vi "KeyboardSimulation_Tests.vi"(11 "error in":errorcluster) -> (15 "error out":errorcluster)   [LabVIEW 2016, in "DronaTest.lvlib"]
uses:
  DronaTest.lvlib
  APIs/Stimulus/KeyBoardSimulation/typedef/VirtualKey.ctl
  APIs/Stimulus/KeyBoardSimulation/typedef/Action.ctl
  APIs/Stimulus/KeyBoardSimulation/KeyBoardSimulationForTargetVI.vi
  APIs/Assert/AssertControlValue/Equal.vi
  <vilib>/addons/_JKI Toolkits/Caraya/classes/Test/Test.lvclass
  Drona.lvlib
  APIs/Stimulus/KeyBoardSimulation/KeyboardSimulation.lvlib
  APIs/Assert/AssertControlValue/AssertControlValue.lvlib
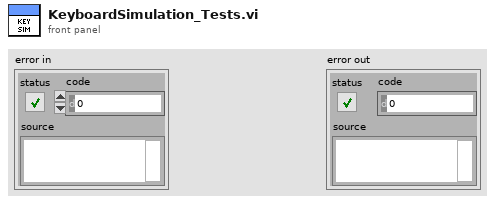
[diagram p1: front panel]
types:
  T1 = typedef "Drona.lvlib/KeyboardSimulation.lvlib/VirtualKey.ctl" = u8
  T2 = typedef "Drona.lvlib/KeyboardSimulation.lvlib/Action.ctl" = enum16{"Press", "Up", "Down"}
  T3 = cluster{" Key":T1, "Action":T2, "Delay (ms)":u32}[]
  T4 = enum16{"TypeHello_ControlValueShouldBeHello", "AddStringToClipboardAndPaste_ControlValueShouldBeStringFromClipboard", "TypeNegative25_ControlValueShouldBeNegative25", "Type255_ControlValueCoerceTo100", "TypeNegative257_ControlValueCoerceToNegative100"}[]
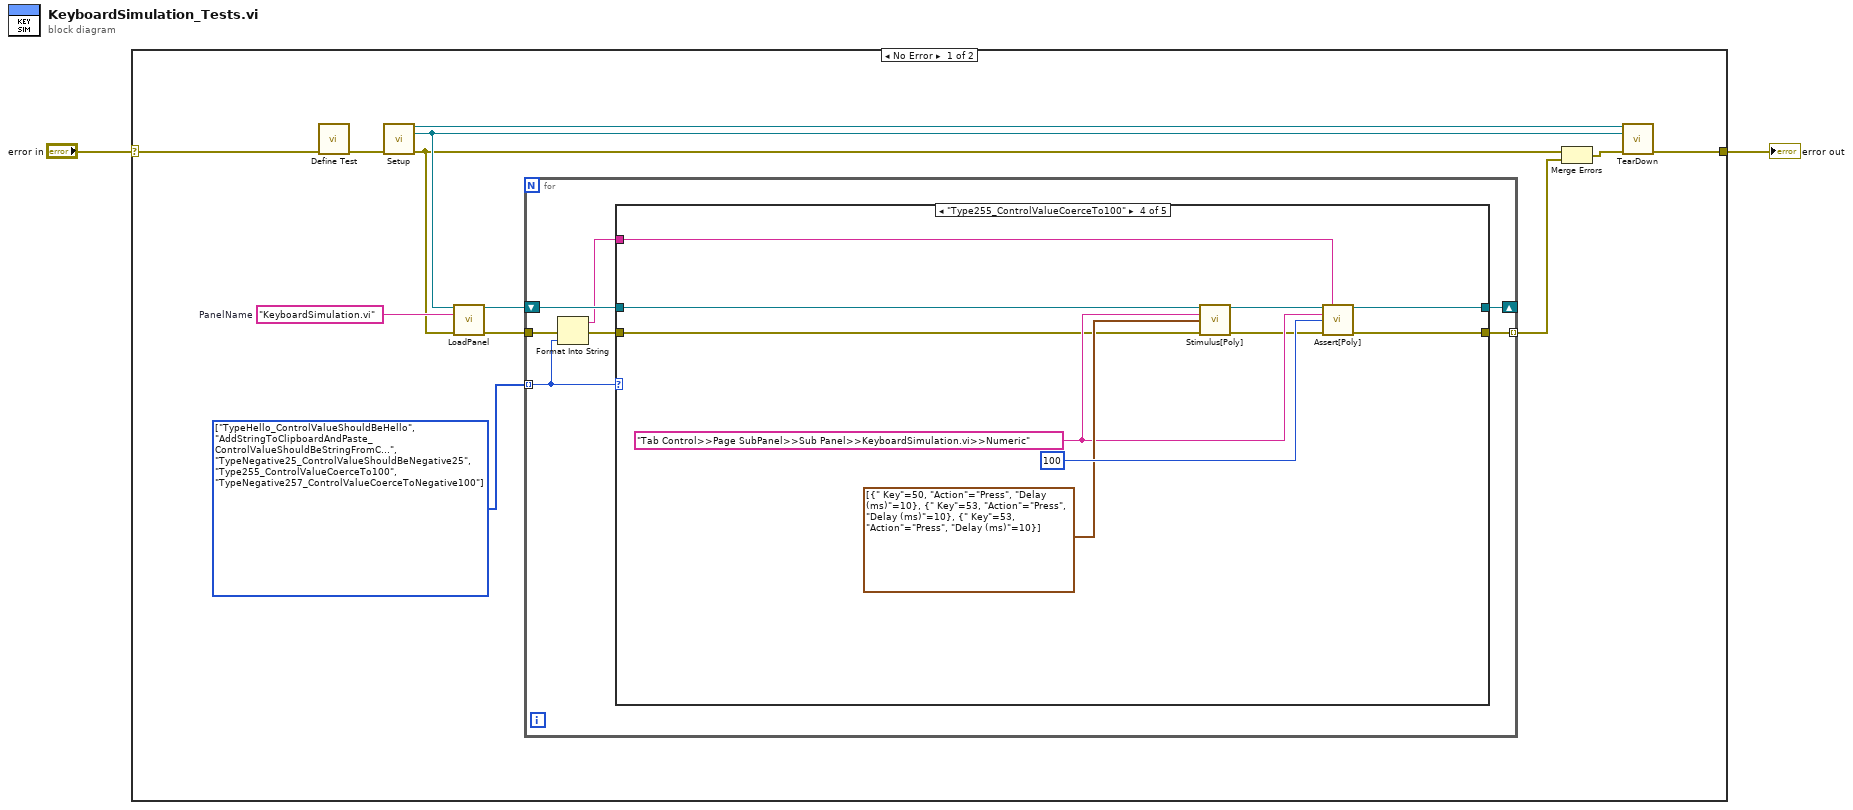
[diagram p0: block diagram]
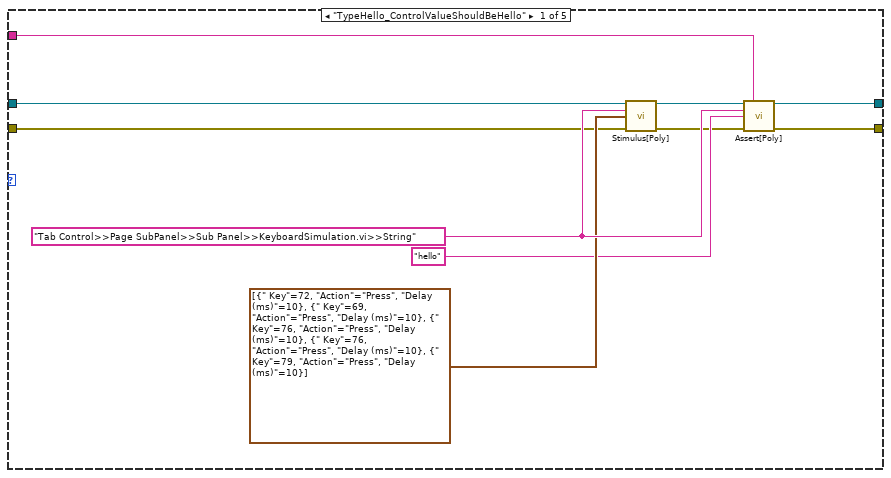
[diagram p2: hidden frame]
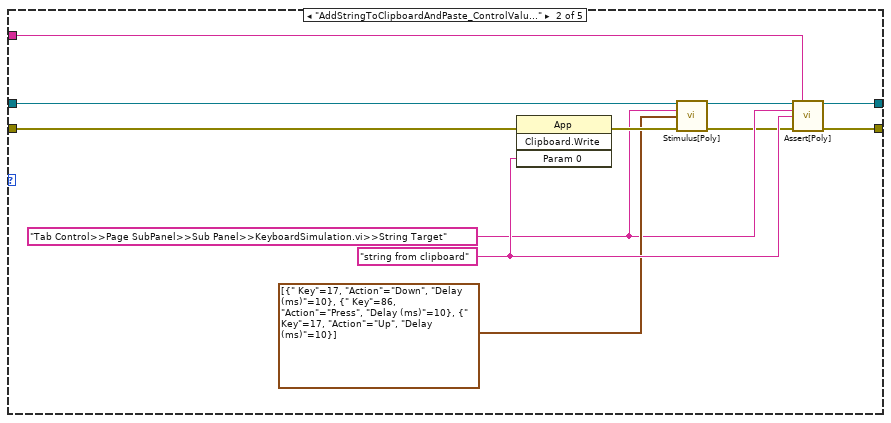
[diagram p3: hidden frame]
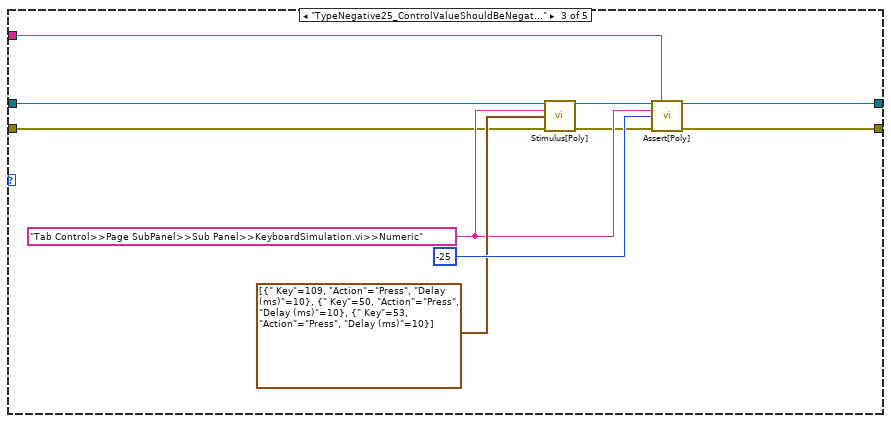
[diagram p4: hidden frame]
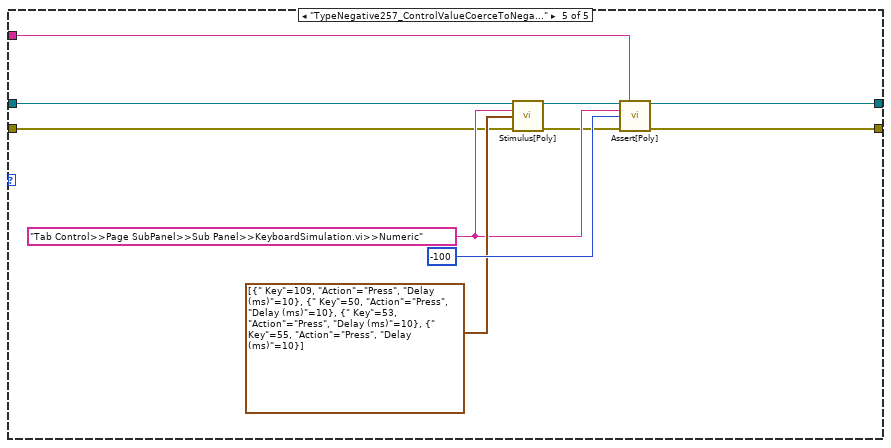
[diagram p5: hidden frame]
diagram:
  n1 = case shown="No Error" "error in" {
    selector: "error in" -> [w14 w73]
    tunnel: [w6 w73] -> w1
    frame No Error {
      w12 = T4 [enum."TypeHello_ControlValueShouldBeHello", enum."AddStringToClipboardAndPaste_ControlValueShouldBeStringFromClipboard", enum."TypeNegative25_ControlValueShouldBeNegative25", enum."Type255_ControlValueCoerceTo100", enum."TypeNegative257_ControlValueCoerceToNegative100"] items=["TypeHello_ControlValueShouldBeHello", "AddStringToClipboardAndPaste_ControlValueShouldBeStringFromClipboard", "TypeNegative25_ControlValueShouldBeNegative25", "Type255_ControlValueCoerceTo100", "TypeNegative257_ControlValueCoerceToNegative100"] ("TestCases")
      w13 = "KeyboardSimulation.vi"  # PanelName
      n2 = call <vilib>:"Define Test.vi"("error in (no error)"=w14) -> ("error out"=w8:errorcluster)  [unwired: 9 in, 1 out]
      n3 = call "Setup.vi"("error in (no error)"=w8) -> ("Application Ref"=w5:refnum<vi>, "VI out"=w4:refnum<vi>, "error out"=w3:errorcluster)  [unwired: 12 in]
      n4 = call "LoadPanel.vi"("VI in"=w4, "Item Name"=w13, "error in (no error)"=w3) -> ("VI out"=w9:refnum<vi>, "error out"=w11:errorcluster)  [unwired: 11 in]
      n5 = for {
        tunnel: w12 -> [w16] mode=indexing
        shift-right: [w20] -> _
        shift-left: w9 -> [w21]
        tunnel: w11 -> [w19]
        tunnel: [w18] -> w10 mode=indexing
        n6 = Format Into String(error in=w19, w16) -> (resulting string=w15:string, error out=w17:errorcluster)  [unwired: 2 in]
        n7 = case shown="\"Type255_ControlValueCoerceTo100\"" w16 {
          tunnel: [w26 w36 w47 w57 w67] -> w18
          tunnel: w21 -> [w25 w34 w45 w55 w65]
          tunnel: [w24 w35 w46 w56 w66] -> w20
          tunnel: w17 -> [w23 w33 w44 w54 w64]
          tunnel: w15 -> [w22 w32 w43 w53 w63]
          frame "TypeHello_ControlValueShouldBeHello" {
            w31 = "Tab Control>>Page SubPanel>>Sub Panel>>KeyboardSimulation.vi>>String" ("Control Path")
            n8 = call-poly "Stimulus[Poly].vi"("VI Reference In"=w25, "Control Path"=w31, "Key Array"=T3 [{" Key"=72, "Action"=enum."Press", "Delay (ms)"=10}, {" Key"=69, "Action"=enum."Press", "Delay (ms)"=10}, {" Key"=76, "Action"=enum."Press", "Delay (ms)"=10}, {" Key"=76, "Action"=enum."Press", "Delay (ms)"=10}, {" Key"=79, "Action"=enum."Press", "Delay (ms)"=10}], "error In"=w23) -> ("VI Reference Out"=w28:refnum<vi>, "error IO"=w27:errorcluster)  [unwired: 10 in]
            n9 = call-poly "Assert[Poly].vi"("VI Reference In"=w28, "Test Label"=w22, "Control Path"=w31, "Control Value"="hello" ("Control Path"), "Error In"=w27) -> ("VI Reference Out"=w24:refnum<vi>, "Error Out"=w26:errorcluster)  [unwired: 8 in, 1 out]
          }
          frame "AddStringToClipboardAndPaste_ControlValueShouldBeStringFromClipboard" {
            w42 = "string from clipboard" ("Control Path")
            w39 = "Tab Control>>Page SubPanel>>Sub Panel>>KeyboardSimulation.vi>>String Target" ("Control Path")
            n10 = invoke on="Invoke Node" class="App" method="Clipboard.Write"(error in=w33, "Param 0"=w42) -> (error out=w41:errorcluster)  [unwired: 2 in, 3 out]
            n11 = call-poly "Stimulus[Poly].vi"("VI Reference In"=w34, "Control Path"=w39, "Key Array"=T3 [{" Key"=17, "Action"=enum."Down", "Delay (ms)"=10}, {" Key"=86, "Action"=enum."Press", "Delay (ms)"=10}, {" Key"=17, "Action"=enum."Up", "Delay (ms)"=10}], "error In"=w41) -> ("VI Reference Out"=w37:refnum<vi>, "error IO"=w38:errorcluster)  [unwired: 10 in]
            n12 = call-poly "Assert[Poly].vi"("VI Reference In"=w37, "Test Label"=w32, "Control Path"=w39, "Control Value"=w42, "Error In"=w38) -> ("VI Reference Out"=w35:refnum<vi>, "Error Out"=w36:errorcluster)  [unwired: 8 in, 1 out]
          }
          frame "TypeNegative25_ControlValueShouldBeNegative25" {
            w50 = "Tab Control>>Page SubPanel>>Sub Panel>>KeyboardSimulation.vi>>Numeric" ("Control Path")
            n13 = call-poly "Stimulus[Poly].vi"("VI Reference In"=w45, "Control Path"=w50, "Key Array"=T3 [{" Key"=109, "Action"=enum."Press", "Delay (ms)"=10}, {" Key"=50, "Action"=enum."Press", "Delay (ms)"=10}, {" Key"=53, "Action"=enum."Press", "Delay (ms)"=10}], "error In"=w44) -> ("VI Reference Out"=w48:refnum<vi>, "error IO"=w49:errorcluster)  [unwired: 10 in]
            n14 = call-poly "Assert[Poly].vi"("VI Reference In"=w48, "Test Label"=w43, "Control Path"=w50, "Control Value"=-25 ("Control Path"), "Error In"=w49) -> ("VI Reference Out"=w46:refnum<vi>, "Error Out"=w47:errorcluster)  [unwired: 8 in, 1 out]
          }
          frame "Type255_ControlValueCoerceTo100" {
            w60 = "Tab Control>>Page SubPanel>>Sub Panel>>KeyboardSimulation.vi>>Numeric" ("Control Path")
            n15 = call-poly "Stimulus[Poly].vi"("VI Reference In"=w55, "Control Path"=w60, "Key Array"=T3 [{" Key"=50, "Action"=enum."Press", "Delay (ms)"=10}, {" Key"=53, "Action"=enum."Press", "Delay (ms)"=10}, {" Key"=53, "Action"=enum."Press", "Delay (ms)"=10}], "error In"=w54) -> ("VI Reference Out"=w58:refnum<vi>, "error IO"=w59:errorcluster)  [unwired: 10 in]
            n16 = call-poly "Assert[Poly].vi"("VI Reference In"=w58, "Test Label"=w53, "Control Path"=w60, "Control Value"=100 ("Control Path"), "Error In"=w59) -> ("VI Reference Out"=w56:refnum<vi>, "Error Out"=w57:errorcluster)  [unwired: 8 in, 1 out]
          }
          frame "TypeNegative257_ControlValueCoerceToNegative100" {
            w70 = "Tab Control>>Page SubPanel>>Sub Panel>>KeyboardSimulation.vi>>Numeric" ("Control Path")
            n17 = call-poly "Stimulus[Poly].vi"("VI Reference In"=w65, "Control Path"=w70, "Key Array"=T3 [{" Key"=109, "Action"=enum."Press", "Delay (ms)"=10}, {" Key"=50, "Action"=enum."Press", "Delay (ms)"=10}, {" Key"=53, "Action"=enum."Press", "Delay (ms)"=10}, {" Key"=55, "Action"=enum."Press", "Delay (ms)"=10}], "error In"=w64) -> ("VI Reference Out"=w68:refnum<vi>, "error IO"=w69:errorcluster)  [unwired: 10 in]
            n18 = call-poly "Assert[Poly].vi"("VI Reference In"=w68, "Test Label"=w63, "Control Path"=w70, "Control Value"=-100 ("Control Path"), "Error In"=w69) -> ("VI Reference Out"=w66:refnum<vi>, "Error Out"=w67:errorcluster)  [unwired: 8 in, 1 out]
          }
        }
      }
      n19 = Merge Errors(w3, w10) -> (w7:errorcluster)
      n20 = call "TearDown.vi"("Application Ref"=w5, "VI in"=w4, "error in (no error)"=w7) -> ("error out"=w6:errorcluster)  [unwired: 12 in]
    }
    frame Error {
    }
  }
  "error out" <- w1
